vi "Compare_odour_components.vi"(0 "Odour component 1":T1, 1 "Proportion 1":cluster{"Numeric":dbl}, 2 "Odour component 2":T1, 3 "Proportion 2":cluster{"Numeric":dbl}, 4 "Odour component data":T2) -> (6 "Distance":dbl)   [LabVIEW 2016]
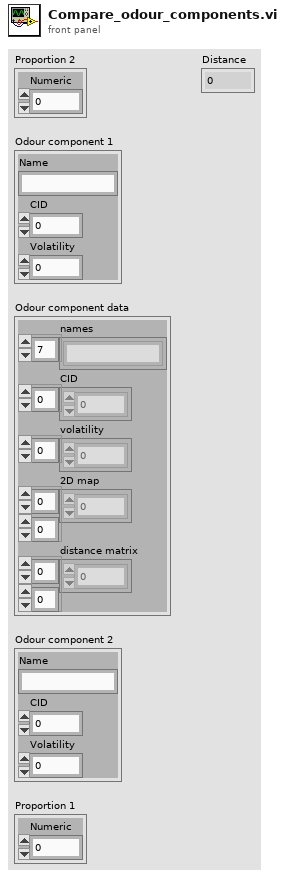
[diagram p1: front panel]
types:
  T1 = cluster{"Name":string, "CID":i32, "Volatility":dbl}
  T2 = cluster{"names":string[], "CID":i32[], "volatility":dbl[], "2D map":dbl[][], "distance matrix":dbl[][]}
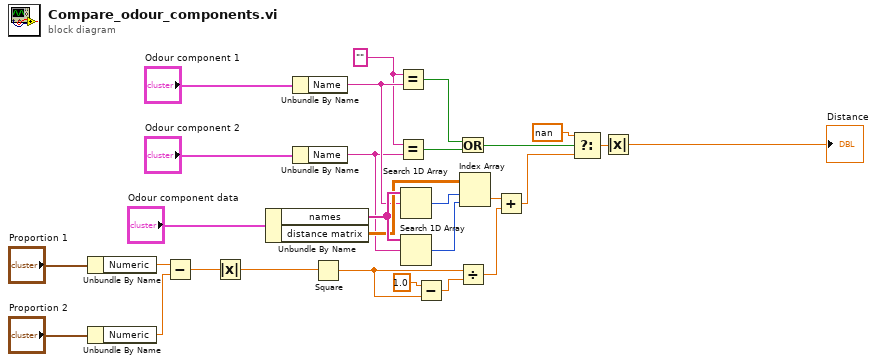
[diagram p0: block diagram]
diagram:
  w9 = "" ("x")
  n1 = Unbundle By Name("Proportion 1") -> ("Numeric"=w15:dbl)
  n2 = Unbundle By Name("Proportion 2") -> ("Numeric"=w16:dbl)
  n3 = Subtract(x=w15, y=w16) -> (x-y=w17:dbl)
  n4 = Absolute Value(x=w17) -> (abs(x)=w19:dbl)
  n5 = Unbundle By Name("Odour component data") -> ("names"=w23:string[], "distance matrix"=w18:dbl[][])
  n6 = Unbundle By Name("Odour component 1") -> ("Name"=w10:string)
  n7 = Unbundle By Name("Odour component 2") -> ("Name"=w8:string)
  n8 = Square(x=w19) -> (x^2=w21:dbl)
  n9 = Equal?(x=w9, y=w10) -> (x = y?=w7:bool)
  n10 = Equal?(x=w9, y=w8) -> (x = y?=w6:bool)
  n11 = Search 1D Array(1D array=w23, element=w10) -> (index of element=w24:i32)  [unwired: 1 in]
  n12 = Search 1D Array(1D array=w23, element=w8) -> (index of element=w25:i32)  [unwired: 1 in]
  n13 = Subtract(x=1.0, y=w21) -> (x-y=w22:dbl)
  n14 = Or(x=w7, y=w6) -> (x .or. y?=w5:bool)
  n15 = Divide(x=w21, y=w22) -> (x/y=w26:dbl)
  n16 = Index Array(array=w18, index (row)=w24, index (col)=w25) -> (element=w27:dbl)
  n17 = Add(x=w27, y=w26) -> (x+y=w4:dbl)
  n18 = Select(t=nan, s=w5, f=w4) -> (s? t:f=w2:dbl)
  n19 = Absolute Value(x=w2) -> (abs(x)=→"Distance":dbl)
